vi "SP - set cluster element.vi"(8 "error in (no error)":errorcluster, 11 "JSON string":string) -> (0 "error out":errorcluster, 3 "value":string)   [LabVIEW 2020, in "ui-testing.lvlib"]
doc: "copyright: Thomas Zilliox©"
uses:
  ui-testing.lvlib
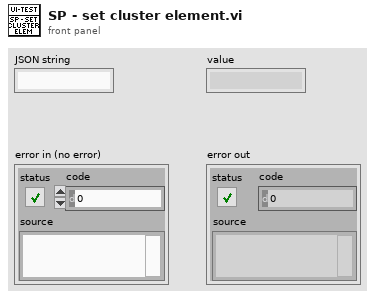
[diagram p1: front panel]
types:
  T1 = cluster{"name":string, "type":string, "value":string, "layers":string[], "subpanel":string}
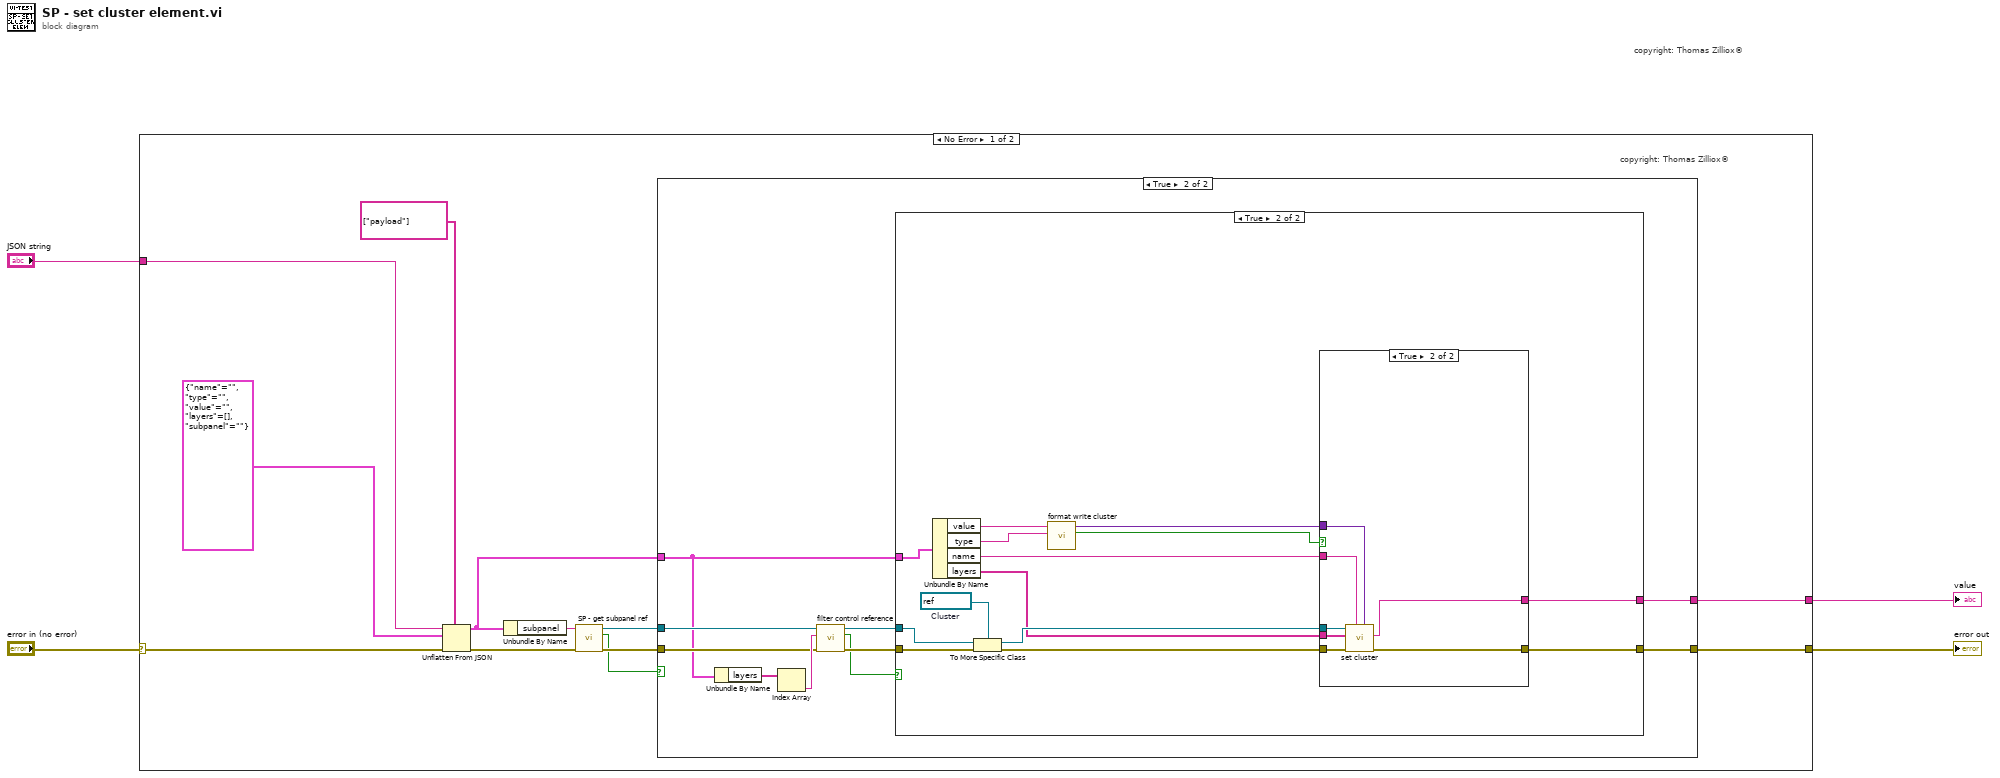
[diagram p0: block diagram]
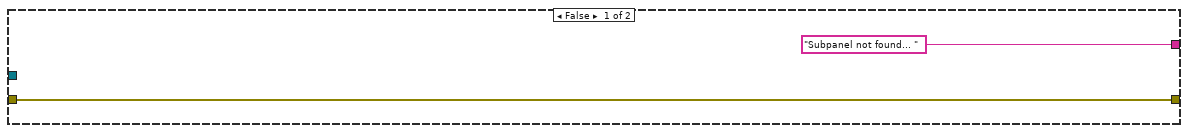
[diagram p2: hidden frame]
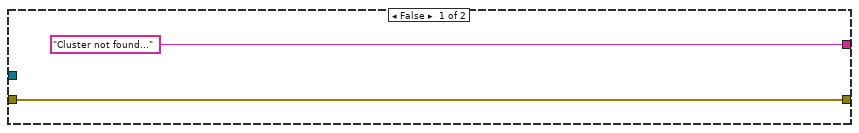
[diagram p3: hidden frame]
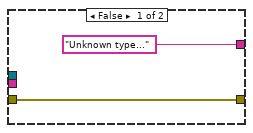
[diagram p4: hidden frame]
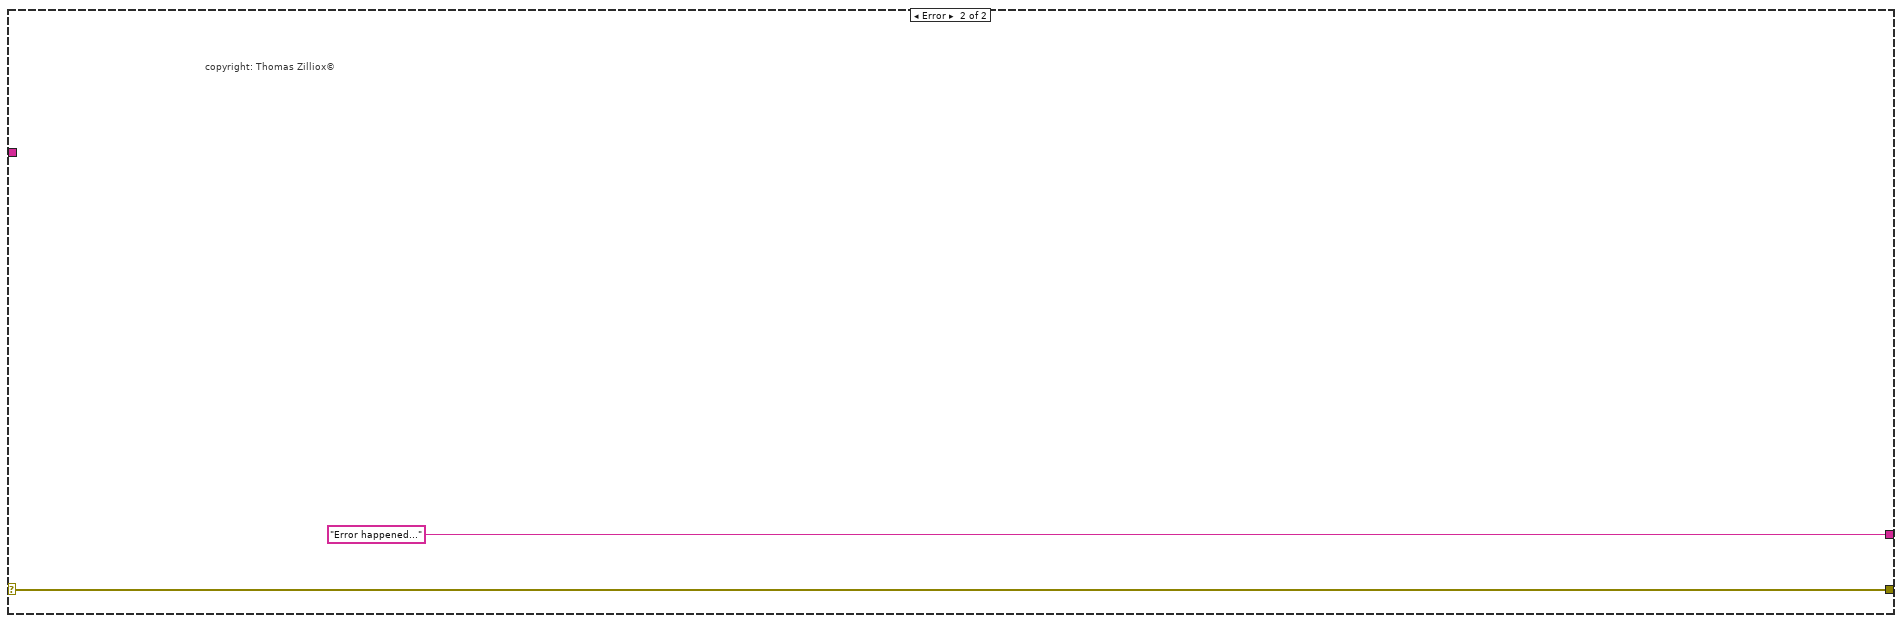
[diagram p5: hidden frame]
diagram:
  # "copyright: Thomas Zilliox©"
  n1 = case shown="No Error" "error in (no error)" {
    selector: "error in (no error)" -> [w14 w55]
    tunnel: "JSON string" -> [w15 _]
    tunnel: [w11 w55] -> w3
    tunnel: [w12 "Error happened..."] -> w2
    frame No Error {
      # "copyright: Thomas Zilliox©"
      n2 = Unflatten From JSON(path=string[] ["payload"], JSON string=w15, type and defaults=T1 {"name"="", "type"="", "value"="", "layers"=[], "subpanel"=""}, error in (no error)=w14) -> (value=w7:T1, error out=w10:errorcluster)  [unwired: 3 in]
      n3 = Unbundle By Name(w7) -> ("subpanel"=w6:string)
      n4 = call "SP - get subpanel ref.vi"("error in (no error)"=w10, "subpanel"=w6) -> ("error out"=w9:errorcluster, "subpanel found ?"=w5:bool, "subpanel VI ref"=w8:refnum<vi>)  [unwired: 6 in, 1 out]
      n5 = case shown="True" w5 {
        tunnel: ["Subpanel not found... " ("result string") w23] -> w12
        tunnel: [w17 w22] -> w11
        tunnel: w9 -> [w17 w21]
        tunnel: w8 -> [_ w20]
        tunnel: w7 -> [_ w19]
        frame False {
        }
        frame True {
          n6 = Unbundle By Name(w19) -> ("layers"=w28:string[])
          n7 = Index Array(array=w28) -> (element=w27:string)  [unwired: 1 in]
          n8 = call "filter control reference.vi"("error in (no error)"=w21, "Control label"=w27, "VI (Caller)"=w20) -> ("error out"=w25:errorcluster, "Control found"=w24:bool, "Control ref"=w26:refnum<vi>)  [unwired: 6 in]
          n9 = case shown="True" w24 {
            tunnel: w26 -> [_ w41]
            tunnel: w25 -> [w30 w44]
            tunnel: [w30 w43] -> w22
            tunnel: ["Cluster not found..." w35] -> w23
            tunnel: w19 -> [_ w38]
            frame False {
            }
            frame True {
              w39 = refnum<vi> refnum  # Cluster
              n10 = Unbundle By Name(w38) -> ("value"=w34:string, "type"=w33:string, "name"=w36:string, "layers"=w37:string[])
              n11 = To More Specific Class(target class=w39, reference=w41, error in=w44) -> (specific class reference=w40:refnum<vi>, error out=w42:errorcluster)
              n12 = call "format write cluster.vi"("type"=w33, "value"=w34) -> ("Valid ?"=w31:bool, "Variant"=w32:variant)  [unwired: 8 in]
              n13 = case shown="True" w31 {
                tunnel: [w46 w53] -> w43
                tunnel: w42 -> [w46 w52]
                tunnel: w40 -> [_ w51]
                tunnel: w37 -> [_ w50]
                tunnel: w36 -> [_ w49]
                tunnel: ["Unknown type..." w47] -> w35
                tunnel: w32 -> [_ w48]
                frame False {
                }
                frame True {
                  n14 = call "set cluster.vi"("Value"=w48, "Label"=w49, "error in (no error)"=w52, "Layer arrary"=w50, "cluster ref"=w51) -> ("error out"=w53:errorcluster, "Acknowledge message"=w47:string)  [unwired: 5 in]
                }
              }
            }
          }
        }
      }
    }
    frame Error {
      # "copyright: Thomas Zilliox©"
    }
  }
  "error out" <- w3
  "value" <- w2
